vi "Frequency from bin number RT.vi"(7 "FFT size":dbl=512.0 format="%#_13g", 10 "Bin number":dbl, 11 "Sample Rate (S/s)":dbl=50000000.0 format="%#_13g") -> (3 "Detected Frequency (Hz)":dbl)   [LabVIEW 2014]
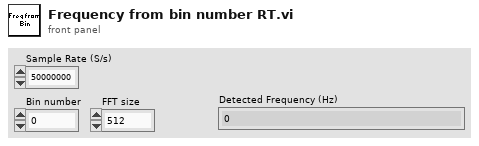
[diagram p1: front panel]
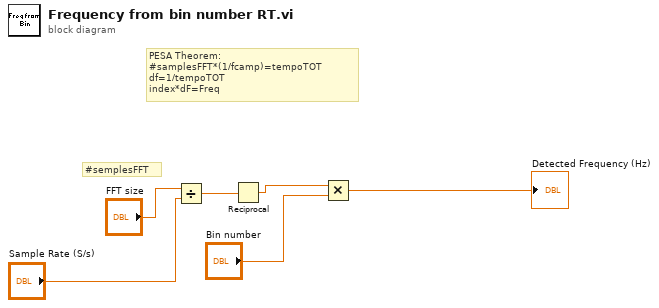
[diagram p0: block diagram]
diagram:
  # "#semplesFFT"
  # "PESA Theorem:\n#samplesFFT*(1/fcamp)=tempoTOT\ndf=1/tempoTOT\nindex*dF=Freq"
  n1 = Divide(x="FFT size", y="Sample Rate (S/s)") -> (x/y=w5:dbl)
  n2 = Reciprocal(x=w5) -> (1/x=w4:dbl)
  n3 = Multiply(x=w4, y="Bin number") -> (x*y=→"Detected Frequency (Hz)":dbl)
